vi "cwave_cachen.vi"(5 "Timing input":path=path "D:/Herbert/MeTimingDLL_test/bin/Release/MOTConf.csv", 10 "Loop number":i16, 11 "Update rate (kHz)":i32=20) -> ()   [LabVIEW 2009]
uses:
  dll.dll
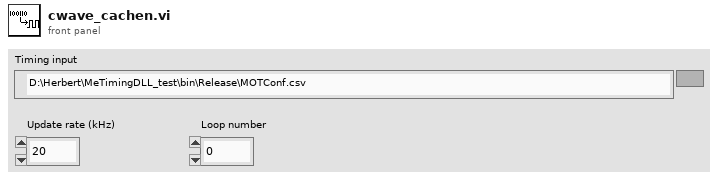
[diagram p1: front panel]
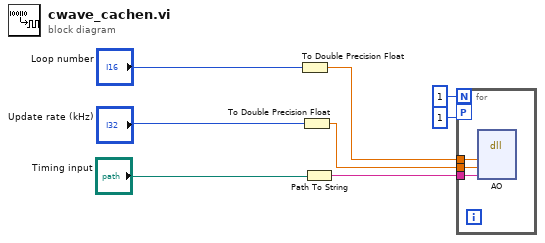
[diagram p0: block diagram]
diagram:
  n1 = To Double Precision Float(number="Loop number") -> (double precision float=w5:dbl)
  n2 = To Double Precision Float(number="Update rate (kHz)") -> (double precision float=w4:dbl)
  n3 = Path To String(path="Timing input") -> (string=w3:string)
  n4 = for {
    N: 1 -> [_]
    tunnel: w5 -> [w11]
    tunnel: w4 -> [w10]
    tunnel: w3 -> [w9]
    workers-P: 1 -> [_]
    n5 = dll-call lib="D:/Herbert/MeTimingDLL_test/bin/Release/dll.dll" fn="AO"("loop"=w11, "sample_rate"=w10, "conf_path"=w9) -> ()  [unwired: 7 in, 2 out]
  }
